vi "Set_Value_Mercury.vi"(8 "error in":errorcluster, 10 "Noun(s)":string, 11 "Mercury Reference In":T1) -> (0 "error out":errorcluster, 3 "Response":string)   [LabVIEW 2019]
uses:
  Public/Controls/Mercury Reference.ctl
  Public/Controls/Comms Transport Layer.ctl
  Private/Controls/Query Dynamic Reference.ctl
  Public/Controls/ISOBus Address.ctl
  Mercury iXX.lvlib
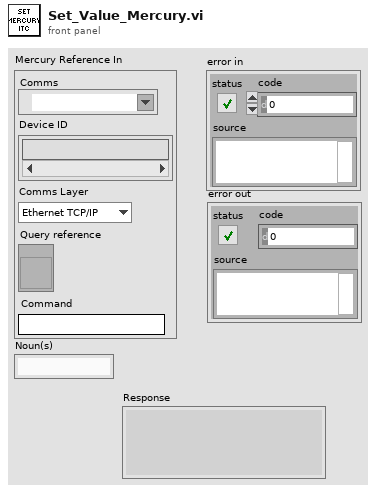
[diagram p1: front panel]
types:
  T1 = typedef "Mercury iXX.lvlib/Mercury Reference.ctl" = cluster{"Comms":refnum<visa-resource-name>, "Device ID":string[], "Comms Layer":T2, "Command":string, "Query reference":T3}
  T2 = typedef "Mercury iXX.lvlib/Comms Transport Layer.ctl" = enum16{"Ethernet TCP/IP", "USB", "ISOBus - RS-232", "GPIB"}
  T3 = typedef "Mercury iXX.lvlib/Query Dynamic Reference.ctl" = refnum<vi>
  T4 = typedef "Mercury iXX.lvlib/ISOBus Address.ctl" = i32
  T5 = typedef "Mercury iXX.lvlib/Response String.ctl" = string
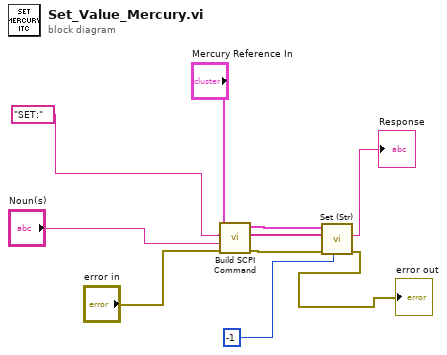
[diagram p0: block diagram]
diagram:
  n1 = call "Build SCPI Command.vi"("error in"="error in", "Noun(s)"="Noun(s)", "Verb"="SET:", "Mercury Reference In"="Mercury Reference In") -> ("error out"=w7:errorcluster, "SCPI Message(s)"=w5:string[], "Mercury Reference Out"=w6:T1)  [unwired: 5 in]
  n2 = call "Set (Str).vi"("ISOBUS address"=T4 -1, "error in"=w7, "SCPI Message(s)"=w5, "Mercury Reference In"=w6) -> ("error out"=→"error out":errorcluster, "Response"=→"Response":T5)  [unwired: 4 in, 2 out]
